vi "HFRR ADV v013 new software.vi"() -> ()   [LabVIEW 2025] (continued)
            frame 2 {
              n1465 = local write "HUMIDITY:"(w1752) -> ()
            }
            frame 3 {
              n1466 = local write "AIR TEMPERATURE :"(w1753) -> ()
            }
            frame 4 {
              n1467 = local write "Com Port 1"(w1754) -> ()
            }
            frame 5 {
              n1468 = local write "Com Port 2"(w1755) -> ()
              n1469 = local write "visa due"(w1755) -> ()
            }
            frame 6 {
              n1470 = String To Path(string=w1756) -> (path=w1757:path)
              n1471 = local write "File Path"(w1757) -> ()
              "String" <- w1756
            }
            frame 7 {
              n1472 = local write "DISPLACEMENT :"(w1758) -> ()
            }
            frame 8 {
              n1473 = local write "STROKE GAIN :"(w1759) -> ()
            }
            frame 9 {
            }
            frame 10 {
              n1474 = local write "Language Selection"(w1760) -> ()
            }
            frame 11 {
              n1475 = local write "CH-POWER +"(w1761) -> ()
            }
            frame 12 {
              n1476 = local write "CH-POWER -"(w1762) -> ()
            }
            frame 13 {
              n1477 = local write "CH-HEATER"(w1763) -> ()
            }
            frame 14 {
              n1478 = local write "CH-HUMIDITY WET"(w1764) -> ()
            }
            frame 15 {
              n1479 = local write "CH-HUMIDITY DRY"(w1765) -> ()
            }
            frame 16 {
            }
            frame 17 {
              n1480 = local write "AIR TEMP INTERCEPT:"(w1766) -> ()
            }
            frame 18 {
              n1481 = local write "TEMP INTERCEPT:"(w1767) -> ()
            }
            frame 21 {
              n1482 = local write "S.NO"(w1768) -> ()
            }
            frame 22 {
              n1483 = local write "Com Port 3"(w1769) -> ()
            }
            frame 20 {
              n1484 = local write "Camera Port :"(w1770) -> ()
            }
            frame 19 {
              n1485 = local write "C3 :"(w1771) -> ()
            }
            frame 23, Default {
            }
          }
        }
      }
    }
    n1486 = Select(t=u32 2500 ("milliseconds to wait"), s=w1724, f=u32 500 ("milliseconds to wait")) -> (s? t:f=w1722:u32)
    n1487 = Multiply(x=w1727, y=w1722) -> (x*y=w1729:dbl)
    n1488 = property on="Time slide" class="Slide (strict)"("Visible"=w1718) -> ()  [unwired: 2 in, 2 out]
    n1489 = call "Elapsed Time2"("Time Target (s)"=w1729, "Auto Reset"=TRUE) -> ("Time has Elapsed"=w1719:bool)  [unwired: 10 in, 7 out]
    n1490 = case shown="True" w1719 {
      frame False {
      }
      frame True {
        n1491 = stacked-sequence {
          frame #0 {
            # "DATA PROCESSING"
            # "115 mV/N"
            n1492 = local read "Sample Temperature"() -> (w1774:dbl)
            n1493 = local read "RH Numeric:"() -> (w1781:dbl)
            n1494 = local read "HUMIDITY:"() -> (w1782:dbl)
            n1495 = local read "FRICVALZ"() -> (w1793:dbl)
            n1496 = local read "Friction"() -> (w1777:dbl)
            n1497 = Multiply(x=w1781, y=w1782) -> (x*y=→"Humidity ( %RH )" →"Hum" →"Hum 2":dbl)
            n1498 = call <vilib>:"Mean PtByPt.vi"("x"=w1774, "sample length"=100) -> ("mean"=w1773:dbl)  [unwired: 2 in, 1 out]
            "TEMP 2" <- w1773
            "TEMP 3" <- w1773
            n1499 = Subtract(x=w1777, y=w1793) -> (x-y=w1788:dbl)
            "FF 2" <- w1788
            "FF 4" <- w1788
            n1500 = local read "Ambient Temperature"() -> (→"AIR TEMP":dbl)
            n1501 = local read "TEMP"() -> (w1792:dbl)
            n1502 = local write "FF 3"(w1788) -> ()
            n1503 = Compound Arithmetic op=OR("FRICVALZ 4", "FRICVALZ 3", "FRICVALZ 2") -> (w1784:bool)
            n1504 = case shown="True" w1784 {
              tunnel: w1777 -> [_ w1799]
              frame False {
              }
              frame True {
                w1798 = FALSE ("FRICVALZ")
                n1505 = local write "FRICVALZ 3"(w1798) -> ()
                n1506 = local write "FRICVALZ 2"(w1798) -> ()
                n1507 = local write "FRICVALZ 4"(w1798) -> ()
                "FRICVALZ" <- w1799
              }
            }
            n1508 = Not A Number/Path/Refnum?(number/path/refnum=w1792) -> (NaN/Path/Refnum?=w1791:bool)
            n1509 = Not A Number/Path/Refnum?(number/path/refnum=w1788) -> (NaN/Path/Refnum?=w1790:bool)
            n1510 = Divide(x=w1788, y=1.96) -> (x/y=w1785:dbl)
            n1511 = Compound Arithmetic op=OR(w1791, w1790) -> (w1789:bool)
            n1512 = Not A Number/Path/Refnum?(number/path/refnum=w1785) -> (NaN/Path/Refnum?=w1786:bool)
            n1513 = case shown="True" w1789 {
              frame False {
              }
              frame True {
                n1514 = local write "TEMP"(0.0 ("TEMP")) -> ()
                n1515 = local write "FF 2"(0.0 ("FF 2")) -> ()
                n1516 = local write "reinit"(TRUE ("reinit")) -> ()
              }
            }
            n1517 = local write "TEMP"(w1773) -> ()
            n1518 = Select(t=0.0, s=w1786, f=w1785) -> (s? t:f=w1776:dbl)
            "COF 2" <- w1776
            n1519 = local write "COF 3"(w1776) -> ()
          }
        }
      }
    }
    n1520 = Wait (ms)(milliseconds to wait=u32 50) -> ()  [unwired: 1 out]
    n1521 = local read "Quit"() -> (w1711:bool)
    "Rate" <- 2500.0 ("No of Samples")
  }
  n1522 = while {
    tunnel: w57 -> [_]
    tunnel: [w1826] -> _
    tunnel: [w1802] -> w56
    i -> [w1826]
    stop <- w1802 stop-if-true
    # "C:\\LAB-IQ-NXT\\Scar View.exe"
    n1523 = local read "OK Button 16"() -> (w1815:bool)
    n1524 = local read "Main Tab"() -> (w1808:T2)
    n1525 = local read "service 3"() -> (w1809:bool)
    n1526 = local read "OPEN 6"() -> (w1811:bool)
    n1527 = local read "EDIT 2"() -> (w1813:bool)
    n1528 = flat-sequence {
      frame #0 {
        n1529 = local read "SAVE 2"() -> (w2428:bool)
        n1530 = stacked-sequence {
          frame #0 {
            n1531 = local read "EDIT"() -> (w2482:bool)
            n1532 = case shown="True" w2482 {
              tunnel: [u8 2 ("Disabled") u8 0 ("Disabled")] -> _
              frame False {
                w2484 = FALSE
                n1533 = local write "Password"("") -> ()
                n1534 = property on="SrvM CP" class="Bool (strict)"("Visible"=w2484) -> ()  [unwired: 2 in, 2 out]
                n1535 = property on="message" class="Str"("Visible"=w2484) -> ()  [unwired: 2 in, 2 out]
                n1536 = local write "x = y?"(w2484) -> ()
                n1537 = property on="Password" class="Str"("Visible"=w2484) -> ()  [unwired: 2 in, 2 out]
                n1538 = property on="ENTER THE NEW PASSWORD" class="Str"("Visible"=w2484) -> ()  [unwired: 2 in, 2 out]
                n1539 = property on="ENTER CURRENT PASSWORD" class="Str"("Visible"=w2484) -> ()  [unwired: 2 in, 2 out]
                n1540 = local write "SrvM CP"(w2484) -> ()
              }
              frame True {
                w2487 = TRUE
                n1541 = property on="SrvM CP" class="Bool (strict)"("Visible"=w2487) -> ()  [unwired: 2 in, 2 out]
                n1542 = property on="Password" class="Str"("Visible"=w2487) -> ()  [unwired: 2 in, 2 out]
              }
            }
            "dipl pwd" <- "@143$\n" ("dipl pwd")
          }
          frame #1 {
            # "Gain password"
            n1543 = String To Byte Array(string="ENTER CURRENT PASSWORD") -> (unsigned byte array=w2492:u8[])
            n1544 = Search 1D Array(1D array=w2492, element=u8 10) -> (index of element=w2495:i32)  [unwired: 1 in]
            n1545 = Index Array(array=w2492, index=w2495) -> (element=w2491:u8)
            n1546 = Equal?(x=w2491, y=10) -> (x = y?=w2489:bool)
            n1547 = case shown="True" w2489 {
              frame False {
                n1548 = property on="ENTER THE NEW PASSWORD" class="Str"("Visible"=FALSE) -> ()  [unwired: 2 in, 2 out]
              }
              frame True {
                # "password"
                # "change password logic"
                n1549 = local read "ENTER CURRENT PASSWORD"() -> (w2508:string)
                n1550 = local read "dipl pwd"() -> (w2502:string)
                n1551 = String To Byte Array(string=w2508) -> (unsigned byte array=w2510:u8[])
                n1552 = String To Byte Array(string=w2502) -> (unsigned byte array=w2503:u8[])
                n1553 = Array Size(array=w2510) -> (size(s)=w2507:i32)
                n1554 = Array Size(array=w2503) -> (size(s)=w2505:i32)
                n1555 = for {
                  N: w2507 -> [_]
                  tunnel: w2510 -> [w2534]
                  tunnel: [w2532] -> w2511 mode=indexing
                  tunnel: w2507 -> [w2526]
                  i -> [w2527]
                  n1556 = Decrement(x=w2526) -> (x-1=w2524:i32)
                  n1557 = Equal?(x=w2527, y=w2524) -> (x = y?=w2525:bool)
                  n1558 = Index Array(array=w2534, index=w2527) -> (element=w2528:u8)
                  n1559 = Number To Decimal String(number=w2528) -> (decimal integer string=w2533:string)  [unwired: 1 in]
                  n1560 = Select(t="", s=w2525, f="\r") -> (s? t:f=w2530:string)
                  n1561 = Concatenate Strings(w2533, w2530) -> (w2532:string)
                }
                n1562 = for {
                  N: w2505 -> [_]
                  tunnel: w2503 -> [w2522]
                  tunnel: [w2520] -> w2504 mode=indexing
                  tunnel: w2505 -> [w2517]
                  i -> [w2518]
                  n1563 = Decrement(x=w2517) -> (x-1=w2516:i32)
                  n1564 = Equal?(x=w2518, y=w2516) -> (x = y?=w2515:bool)
                  n1565 = Index Array(array=w2522, index=w2518) -> (element=w2521:u8)
                  n1566 = Number To Decimal String(number=w2521) -> (decimal integer string=w2519:string)  [unwired: 1 in]
                  n1567 = Select(t="", s=w2515, f="\r") -> (s? t:f=w2512:string)
                  n1568 = Concatenate Strings(w2519, w2512) -> (w2520:string)
                }
                n1569 = local read "string"() -> (w2509:string)
                n1570 = Concatenate Strings(w2504) -> (w2498:string)
                n1571 = Concatenate Strings(w2509) -> (w2506:string)
                n1572 = Concatenate Strings(w2511) -> (w2499:string)
                n1573 = Equal?(x=w2499, y=w2506) -> (x = y?=w2501:bool)
                n1574 = Equal?(x=w2499, y=w2498) -> (x = y?=w2497:bool)
                n1575 = Or(x=w2501, y=w2497) -> (x .or. y?=w2500:bool)
                n1576 = case shown="True" w2500 {
                  frame False {
                  }
                  frame True {
                    n1577 = property on="ENTER THE NEW PASSWORD" class="Str"("Visible"=TRUE) -> ()  [unwired: 2 in, 2 out]
                  }
                }
              }
            }
          }
          frame #2 {
            n1578 = String To Byte Array(string="ENTER THE NEW PASSWORD") -> (unsigned byte array=w2537:u8[])
            n1579 = Search 1D Array(1D array=w2537, element=u8 10) -> (index of element=w2541:i32)  [unwired: 1 in]
            n1580 = Index Array(array=w2537, index=w2541) -> (element=w2539:u8)
            n1581 = Equal?(x=w2539, y=10) -> (x = y?=w2536:bool)
            n1582 = case shown="False" w2536 {
              frame False {
              }
              frame True {
                n1583 = local write "EDIT"(FALSE) -> ()
                n1584 = local write "SrvM CP"(FALSE) -> ()
                n1585 = local read "ENTER THE NEW PASSWORD"() -> (w2544:string)
                n1586 = String To Byte Array(string=w2544) -> (unsigned byte array=w2549:u8[])
                n1587 = Array Size(array=w2549) -> (size(s)=w2546:i32)
                n1588 = for {
                  N: w2546 -> [_]
                  tunnel: w2549 -> [w2562]
                  tunnel: [w2559] -> w2551 mode=indexing
                  tunnel: w2546 -> [w2554]
                  i -> [w2552]
                  n1589 = Decrement(x=w2554) -> (x-1=w2555:i32)
                  n1590 = Equal?(x=w2552, y=w2555) -> (x = y?=w2556:bool)
                  n1591 = Index Array(array=w2562, index=w2552) -> (element=w2561:u8)
                  n1592 = Number To Decimal String(number=w2561) -> (decimal integer string=w2560:string)  [unwired: 1 in]
                  n1593 = Select(t="", s=w2556, f="\r") -> (s? t:f=w2553:string)
                  n1594 = Concatenate Strings(w2560, w2553) -> (w2559:string)
                }
                n1595 = local read "file path"() -> (w2543:path)
                n1596 = Concatenate Strings(w2551) -> (w2545:string)
                n1597 = Delete(path (use dialog)=w2543) -> (deleted path=w2547:path)  [unwired: 4 in, 2 out]
                n1598 = call <vilib>:"Write Characters To File.vi"("append to file? (new file:F)"=FALSE, "character string"=w2545, "file path (dialog if empty)"=w2547) -> ()  [unwired: 2 in, 1 out]
              }
            }
          }
          frame #3 {
            n1599 = case shown="True" "SrvM CP" {
              frame False {
                w2565 = ""
                n1600 = local write "ENTER CURRENT PASSWORD"(w2565) -> ()
                n1601 = local write "ENTER THE NEW PASSWORD"(w2565) -> ()
                n1602 = property on="ENTER CURRENT PASSWORD" class="Str"("Visible"=FALSE) -> ()  [unwired: 2 in, 2 out]
              }
              frame True {
                n1603 = property on="ENTER THE NEW PASSWORD" class="Str"() -> ("Visible"=w2566:bool)  [unwired: 2 in, 2 out]
                n1604 = Not(x=w2566) -> (.not. x?=w2567:bool)
                n1605 = property on="ENTER CURRENT PASSWORD" class="Str"("Visible"=w2567) -> ()  [unwired: 2 in, 2 out]
              }
            }
          }
          frame #4 {
            n1606 = String To Byte Array(string="Password") -> (unsigned byte array=w2574:u8[])
            n1607 = Search 1D Array(1D array=w2574, element=u8 10) -> (index of element=w2572:i32)  [unwired: 1 in]
            n1608 = Index Array(array=w2574, index=w2572) -> (element=w2573:u8)
            n1609 = Equal?(x=w2573, y=10) -> (x = y?=w2569:bool)
            n1610 = case shown="True" w2569 {
              frame False {
              }
              frame True {
                # "password"
                # "password"
                n1611 = local read "Password"() -> (w2587:string)
                n1612 = String To Byte Array(string=w2587) -> (unsigned byte array=w2590:u8[])
                n1613 = String To Byte Array(string="@143$\n") -> (unsigned byte array=w2576:u8[])
                n1614 = Array Size(array=w2590) -> (size(s)=w2585:i32)
                n1615 = Array Size(array=w2576) -> (size(s)=w2581:i32)
                n1616 = for {
                  N: w2585 -> [_]
                  tunnel: w2590 -> [w2624]
                  tunnel: [w2622] -> w2591 mode=indexing
                  tunnel: w2585 -> [w2619]
                  i -> [w2620]
                  n1617 = Decrement(x=w2619) -> (x-1=w2618:i32)
                  n1618 = Index Array(array=w2624, index=w2620) -> (element=w2623:u8)
                  n1619 = Equal?(x=w2620, y=w2618) -> (x = y?=w2617:bool)
                  n1620 = Number To Decimal String(number=w2623) -> (decimal integer string=w2621:string)  [unwired: 1 in]
                  n1621 = Select(t="", s=w2617, f="\r") -> (s? t:f=w2614:string)
                  n1622 = Concatenate Strings(w2621, w2614) -> (w2622:string)
                }
                n1623 = for {
                  N: w2581 -> [_]
                  tunnel: w2576 -> [w2635]
                  tunnel: [w2633] -> w2579 mode=indexing
                  tunnel: w2581 -> [w2630]
                  i -> [w2631]
                  n1624 = Decrement(x=w2630) -> (x-1=w2629:i32)
                  n1625 = Index Array(array=w2635, index=w2631) -> (element=w2634:u8)
                  n1626 = Equal?(x=w2631, y=w2629) -> (x = y?=w2628:bool)
                  n1627 = Number To Decimal String(number=w2634) -> (decimal integer string=w2632:string)  [unwired: 1 in]
                  n1628 = Select(t="", s=w2628, f="\r") -> (s? t:f=w2625:string)
                  n1629 = Concatenate Strings(w2632, w2625) -> (w2633:string)
                }
                n1630 = local read "file path"() -> (w2575:path)
                n1631 = call <vilib>:"Read Characters From File.vi"("file path (dialog if empty)"=w2575) -> ("character string"=w2589:string)  [unwired: 5 in, 3 out]
                "string" <- w2589
                n1632 = flat-sequence {
                  tunnel: [w2592] -> w2586
                  frame #0 {
                    w2592 = ""
                    n1633 = local write "Password"(w2592) -> ()
                  }
                }
                n1634 = Concatenate Strings(w2579) -> (w2580:string)
                n1635 = Concatenate Strings(w2589) -> (w2588:string)
                n1636 = Concatenate Strings(w2591) -> (w2583:string)
                n1637 = Equal?(x=w2583, y=w2588) -> (x = y?=w2578:bool)
                n1638 = Equal?(x=w2583, y=w2580) -> (x = y?=w2584:bool)
                n1639 = Or(x=w2578, y=w2584) -> (x .or. y?=w2577:bool)
                "x = y?" <- w2577
                n1640 = case shown="True" w2577 {
                  selector: w2577 -> [w2594 _]
                  tunnel: w2586 -> [_ _]
                  frame False {
                    n1641 = And(x=w2594, y=TRUE ("Visible")) -> (x .and. y?=w2595:bool)
                    n1642 = property on="message" class="Str"("Visible"=w2595) -> ()  [unwired: 2 in, 2 out]
                  }
                  frame True {
                    n1643 = control-ref of="This VI"() -> (w2606:refnum<vi>)
                    n1644 = property class="VI"(reference=w2606) -> (reference out=w2597:refnum<vi>, error out=w2601:errorcluster, "Panel"=w2605:refnum<vi>)  [unwired: 1 in]
                    n1645 = property on="message" class="Str"("Visible"=FALSE) -> ()  [unwired: 2 in, 2 out]
                    n1646 = property class="Pnl"(reference=w2605, error in=w2601) -> (reference out=w2599:refnum<vi>, error out=w2602:errorcluster, "Panes[]"=w2604:refnum<vi>[])
                    n1647 = for {
                      tunnel: w2604 -> [w2613] mode=indexing
                      tunnel: T20."Always On" ("Horizontal Scrollbar Visibility") -> [w2612]
                      tunnel: w2602 -> [w2609]
                      tunnel: [w2608] -> w2600
                      n1648 = property class="Pane"(reference=w2613, error in=w2609, "HorizScrollbarVisibility"=w2612) -> (reference out=w2610:refnum<vi>, error out=w2611:errorcluster)
                      n1649 = Close Reference(reference=w2610, error in (no error)=w2611) -> (error out=w2608:errorcluster)
                    }
                    n1650 = Close Reference(reference=w2599, error in (no error)=w2600) -> (error out=w2598:errorcluster)
                    n1651 = Close Reference(reference=w2597, error in (no error)=w2598) -> (error out=→"error out 6":errorcluster)
                  }
                }
              }
            }
          }
        }
        n1652 = local read "x = y?"() -> (w2434:bool)
        n1653 = local read "HUMIDITY: 2"() -> (w2436:dbl)
        n1654 = local read "HUMIDITY:"() -> (w2435:dbl)
        n1655 = property on="Port 2 Error" class="Clust (strict)"("Visible"="EDIT") -> ()  [unwired: 2 in, 2 out]
        n1656 = property on="Port 1 Error" class="Clust (strict)"("Visible"="EDIT") -> ()  [unwired: 2 in, 2 out]
        n1657 = case shown="True" "SrvM CP 2" {
          frame False {
          }
          frame True {
            n1658 = local write "SrvM CP 2"(FALSE ("SrvM CP 2")) -> ()
            n1659 = local read "HUMIDITY: 2"() -> (w2475:dbl)
            n1660 = local read "TEMP INTERCEPT: 2"() -> (w2474:dbl)
            n1661 = local read "DISPLACEMENT : 4"() -> (w2478:dbl)
            n1662 = local read "TEMPERATURE : 2"() -> (w2477:dbl)
            n1663 = local read "STROKE GAIN : 2"() -> (w2479:dbl)
            n1664 = local read "FRIC. FORCE : 2"() -> (w2480:dbl)
            n1665 = local read "AIR TEMP INTERCEPT: 2"() -> (w2473:dbl)
            n1666 = local read "AIR TEMPERATURE : 2"() -> (w2476:dbl)
            n1667 = local write "HUMIDITY:"(w2475) -> ()
            n1668 = local write "AIR TEMP INTERCEPT:"(w2474) -> ()
            n1669 = local write "TEMPERATURE :"(w2477) -> ()
            n1670 = local write "FRIC. FORCE :"(w2480) -> ()
            n1671 = local write "STROKE GAIN :"(w2479) -> ()
            n1672 = local write "DISPLACEMENT :"(w2478) -> ()
            n1673 = local write "AIR TEMPERATURE :"(w2476) -> ()
            n1674 = local write "TEMP INTERCEPT:"(w2473) -> ()
          }
        }
        n1675 = Or(x="SAVE", y=w2428) -> (x .or. y?=w2429:bool)
        n1676 = And(x="EDIT", y=w2434) -> (x .and. y?=w2432:bool)
        n1677 = local read "DISPLACEMENT : 4"() -> (w2445:dbl)
        n1678 = local read "TEMPERATURE : 2"() -> (w2443:dbl)
        n1679 = local read "STROKE GAIN : 2"() -> (w2449:dbl)
        n1680 = local read "DISPLACEMENT :"() -> (w2444:dbl)
        n1681 = local read "FRIC. FORCE : 2"() -> (w2452:dbl)
        n1682 = local read "TEMPERATURE :"() -> (w2441:dbl)
        n1683 = local read "STROKE GAIN :"() -> (w2448:dbl)
        n1684 = local read "FRIC. FORCE :"() -> (w2451:dbl)
        n1685 = case shown="True" w2432 {
          tunnel: [u8 2 ("Disabled") u8 0 ("Disabled")] -> w2431
          tunnel: [w2796 TRUE ("Visible")] -> w2430
          frame False {
            w2796 = FALSE ("Visible")
            n1686 = local write "EDIT 2"(w2796) -> ()
          }
          frame True {
          }
        }
        n1687 = case shown="True" w2429 {
          frame False {
          }
          frame True {
            n1688 = stacked-sequence {
              seq-local: [w2644 _ _] -> [_ w2791 _]
              frame #0 {
                (unwired) i16 5 ("precision (6)")
                # "[CH1]    - FF\n[CH2]   - TEMPERATURE\n[CH3]    - Humidity\n[CH4]    - AIR TEMP\n[CH5]\\- Visa Uno\n[CH6] \\- Visa Due\n[CH7]  \\- file path\n[CH8]   - Displacement Gain\n[CHA]   - Stroke Gain\n[CHB]   - Stroke PID Gain\n[CHC]   -Language Selection\n[CHD]   -Power +\n[CHE]   -Power_\n[CHF]   -Heater\n[CHG]   -Humidity Wet\n[CHH]   -Humidity Dry\n[CHI]   -Integral Time"
                n1689 = local read "Language Selection"() -> (w2692:enum16{"English", "Russian"})
                n1690 = local read "CH-HUMIDITY WET"() -> (w2650:u16)
                n1691 = local read "CH-HUMIDITY DRY"() -> (w2647:u16)
                n1692 = local read "STROKE GAIN :"() -> (w2636:dbl)
                n1693 = local read "CH-POWER +"() -> (w2659:u16)
                n1694 = local read "CH-POWER -"() -> (w2656:u16)
                n1695 = local read "CH-HEATER"() -> (w2653:u16)
                n1696 = local read "AIR TEMPERATURE :"() -> (w2639:dbl)
                n1697 = local read "DISPLACEMENT :"() -> (w2637:dbl)
                n1698 = local read "TEMPERATURE :"() -> (w2640:dbl)
                n1699 = local read "FRIC. FORCE :"() -> (w2641:dbl)
                n1700 = local read "HUMIDITY:"() -> (w2638:dbl)
                n1701 = Path To String(path="File Path") -> (string=w2708:string)
                n1702 = Number To Fractional String(number=w2636, width (-)=i16 10 ("precision (6)"), precision (6)=i16 5) -> (F-format string=w2699:string)  [unwired: 1 in]
                n1703 = Number To Fractional String(number=w2692, width (-)=i16 10 ("precision (6)"), precision (6)=i16 5) -> (F-format string=w2688:string)  [unwired: 1 in]
                n1704 = Number To Fractional String(number=w2659, width (-)=i16 10 ("precision (6)"), precision (6)=i16 5) -> (F-format string=w2682:string)  [unwired: 1 in]
                n1705 = Number To Fractional String(number=w2656, width (-)=i16 10 ("precision (6)"), precision (6)=i16 5) -> (F-format string=w2679:string)  [unwired: 1 in]
                n1706 = Number To Fractional String(number=w2653, width (-)=i16 10 ("precision (6)"), precision (6)=i16 5) -> (F-format string=w2674:string)  [unwired: 1 in]
                n1707 = Number To Fractional String(number=w2650, width (-)=i16 10 ("precision (6)"), precision (6)=i16 5) -> (F-format string=w2671:string)  [unwired: 1 in]
                n1708 = Number To Fractional String(number=w2647, width (-)=i16 10 ("precision (6)"), precision (6)=i16 5) -> (F-format string=w2666:string)  [unwired: 1 in]
                n1709 = local read "Com Port 1"() -> (w2643:refnum<visa-resource-name>)
                n1710 = local read "Com Port 2"() -> (w2642:refnum<visa-resource-name>)
                n1711 = Concatenate Strings(w2708, "\\" ("string")) -> (w2707:string)
                n1712 = Number To Fractional String(number=w2641, width (-)=i16 10 ("precision (6)"), precision (6)=i16 5) -> (F-format string=w2740:string)  [unwired: 1 in]
                n1713 = Number To Fractional String(number=w2640, width (-)=i16 10 ("precision (6)"), precision (6)=i16 5) -> (F-format string=w2739:string)  [unwired: 1 in]
                n1714 = Number To Fractional String(number=w2638, width (-)=i16 10 ("precision (6)"), precision (6)=i16 5) -> (F-format string=w2733:string)  [unwired: 1 in]
                n1715 = Number To Fractional String(number=w2639, width (-)=i16 10 ("precision (6)"), precision (6)=i16 5) -> (F-format string=w2727:string)  [unwired: 1 in]
                n1716 = Number To Fractional String(number=w2637, width (-)=i16 10 ("precision (6)"), precision (6)=i16 5) -> (F-format string=w2700:string)  [unwired: 1 in]
                n1717 = Concatenate Strings("[CHA]" ("string"), w2699, "- Stroke Gain" ("string"), "\r") -> (w2693:string)
                n1718 = Concatenate Strings("[CHC]" ("string"), w2688, "-Language Selection" ("string"), "\r") -> (w2685:string)
                n1719 = Concatenate Strings("[CHD]" ("string"), w2682, "-Power +" ("string"), "\r") -> (w2664:string)
                n1720 = Concatenate Strings("[CHG]" ("string"), w2671, "-Humidity Wet" ("string"), "\r") -> (w2661:string)
                n1721 = Concatenate Strings("[CHH]" ("string"), w2666, "-Humidity Dry" ("string"), "\r") -> (w2660:string)
                n1722 = Concatenate Strings("[CH1]" ("string"), w2740, " - FF" ("string"), "\r") -> (w2738:string)
                n1723 = Concatenate Strings("[CH2]" ("string"), w2739, " - TEMPERATURE" ("string"), "\r") -> (w2737:string)
                n1724 = Concatenate Strings("[CH3]" ("string"), w2733, " - Humidity" ("string"), "\r") -> (w2730:string)
                n1725 = Concatenate Strings("[CH4]" ("string"), w2727, " - AIR TEMP" ("string"), "\r") -> (w2723:string)
                n1726 = Concatenate Strings("[CH5]" ("string"), w2643, "- Visa Uno" ("string"), "\r") -> (w2716:string)
                n1727 = Concatenate Strings("[CH6]" ("string"), w2642, "- Visa Due" ("string"), "\r") -> (w2711:string)
                n1728 = Concatenate Strings("[CH7]" ("string"), w2707, "- file path" ("string"), "\r") -> (w2710:string)
                n1729 = Concatenate Strings("[CH8]" ("string"), w2700, "- Displacement Gain" ("string"), "\r") -> (w2703:string)
                n1730 = Concatenate Strings("[CHE]" ("string"), w2679, "-Power_" ("string"), "\r") -> (w2663:string)
                n1731 = Concatenate Strings("[CHF]" ("string"), w2674, "-Heater" ("string"), "\r") -> (w2662:string)
                n1732 = Concatenate Strings(w2738, w2737, w2730, w2723, w2716, w2711, w2710, w2703, w2693, w2685, w2664, w2663, w2662, w2661, w2660) -> (w2644:string)
                "gain" <- w2644
              }
              frame #1 {
                n1733 = local read "Camera Port :"() -> (w2752:string)
                n1734 = local read "C3 :"() -> (w2760:refnum<visa-resource-name>)
                n1735 = local read "TEMP INTERCEPT:"() -> (w2761:dbl)
                n1736 = local read "AIR TEMP INTERCEPT:"() -> (w2762:dbl)
                n1737 = local read "Com Port 3"() -> (w2763:refnum<visa-resource-name>)
                n1738 = Concatenate Strings("[CH8]" ("string"), w2752, "- Visa Camera" ("string"), "\r") -> (w2751:string)
                n1739 = Concatenate Strings("[CH7]" ("string"), w2760, "- Visa Humidity" ("string"), "\r") -> (w2756:string)
                n1740 = Number To Fractional String(number=w2761, width (-)=i16 10 ("precision (6)"), precision (6)=i16 5) -> (F-format string=w2779:string)  [unwired: 1 in]
                n1741 = Concatenate Strings("[CHL]" ("string"), w2763, "- Visa humid" ("string"), "\r") -> (w2766:string)
                n1742 = Number To Fractional String(number=w2762, width (-)=i16 10 ("precision (6)"), precision (6)=i16 5) -> (F-format string=w2786:string)  [unwired: 1 in]
                n1743 = Concatenate Strings("[CHK]" ("string"), w2779, "-TEMP INTERCEPT" ("string"), "\r") -> (w2775:string)
                n1744 = Concatenate Strings("[SNO]" ("string"), "S.NO", "-" ("string"), "\r") -> (w2771:string)
                n1745 = Concatenate Strings("[CHJ]" ("string"), w2786, "-AIR TEMP INTERCEPT" ("string"), "\r") -> (w2776:string)
                n1746 = String To Path(string="C:\\LAB-IQ\\calibrate WO 2465.dcf") -> (path=w2764:path)
                n1747 = Concatenate Strings(w2791, w2776, w2775, w2771, w2766, w2756, w2751) -> (w2790:string)
                n1748 = call <vilib>:"Write Characters To File.vi"("append to file? (new file:F)"=FALSE, "character string"=w2790, "file path (dialog if empty)"=w2764) -> ()  [unwired: 2 in, 1 out]
              }
              frame #2 {
                n1749 = local write "Lan flag"(0.0 ("Lan flag")) -> ()
                n1750 = local write "conststatus"(0.0 ("rpm value : 2")) -> ()
                n1751 = local write "SAVE"(FALSE ("OK Button 14")) -> ()
                n1752 = local write "SAVE 2"(FALSE ("SAVE 2")) -> ()
              }
            }
          }
        }
        n1753 = Subtract(x=w2436, y=w2435) -> (x-y=w2437:dbl)
        n1754 = local read "AIR TEMPERATURE : 2"() -> (w2440:dbl)
        n1755 = local read "AIR TEMPERATURE :"() -> (w2439:dbl)
        n1756 = Divide(x=w2437, y=w2435) -> (x/y=w2459:dbl)
        n1757 = Subtract(x=w2452, y=w2451) -> (x-y=w2450:dbl)
        n1758 = Subtract(x=w2443, y=w2441) -> (x-y=w2442:dbl)
        n1759 = Subtract(x=w2449, y=w2448) -> (x-y=w2447:dbl)
        n1760 = Subtract(x=w2445, y=w2444) -> (x-y=w2446:dbl)
        n1761 = Subtract(x=w2440, y=w2439) -> (x-y=w2438:dbl)
        n1762 = Divide(x=w2450, y=w2451) -> (x/y=w2470:dbl)
        n1763 = Divide(x=w2442, y=w2441) -> (x/y=w2463:dbl)
        n1764 = Divide(x=w2447, y=w2448) -> (x/y=w2467:dbl)
        n1765 = Divide(x=w2446, y=w2444) -> (x/y=w2466:dbl)
        n1766 = Multiply(x=w2459, y=100.0) -> (x*y=→"HUMIDITY  Calibration Error":dbl)
        n1767 = Divide(x=w2438, y=w2439) -> (x/y=w2462:dbl)
        n1768 = Multiply(x=w2470, y=100.0) -> (x*y=→"FRIC. FORCE Calibration Error":dbl)
        n1769 = Multiply(x=w2463, y=100.0) -> (x*y=→"TEMPERATURE  Calibration Error":dbl)
        n1770 = Multiply(x=w2467, y=100.0) -> (x*y=→"STROKE Calibration Error":dbl)
        n1771 = Multiply(x=w2466, y=100.0) -> (x*y=→"DISPLACEMENT  Calibration Error":dbl)
        n1772 = property on="EDIT 2" class="Bool (strict)"("Visible"=w2430) -> ()  [unwired: 2 in, 2 out]
        n1773 = property on="SAVE" class="Bool (strict)"("Visible"=w2430) -> ()  [unwired: 2 in, 2 out]
        n1774 = property on="SrvM CP" class="Bool (strict)"("Disabled"=w2431) -> ()  [unwired: 2 in, 2 out]
        n1775 = property on="visa due" class="CmbBox"("Disabled"=w2431) -> ()  [unwired: 2 in, 2 out]
        n1776 = property on="File Path" class="Path"("Disabled"=w2431) -> ()  [unwired: 2 in, 2 out]
        n1777 = Multiply(x=w2462, y=100.0) -> (x*y=→"AIR TEMPERATURE  Calibration Error":dbl)
        n1778 = property on="Language Selection" class="Enum (strict)"("Visible"=w2430) -> ()  [unwired: 2 in, 2 out]
        n1779 = property on="Tab Control 7" class="TabCtl (strict)"("Disabled"=w2431) -> ()  [unwired: 2 in, 2 out]
        n1780 = property on="AIR TEMP INTERCEPT:" class="DigNum (strict)"("Disabled"=w2431) -> ()  [unwired: 2 in, 2 out]
        n1781 = property on="CH-POWER -" class="DigNum (strict)"("Disabled"=w2431) -> ()  [unwired: 2 in, 2 out]
        n1782 = property on="CH-POWER +" class="DigNum (strict)"("Disabled"=w2431) -> ()  [unwired: 2 in, 2 out]
        n1783 = property on="AIR TEMPERATURE :" class="DigNum (strict)"("Disabled"=w2431) -> ()  [unwired: 2 in, 2 out]
        n1784 = property on="STROKE GAIN :" class="DigNum (strict)"("Disabled"=w2431) -> ()  [unwired: 2 in, 2 out]
        n1785 = property on="SPEED OUT:" class="DigNum (strict)"("Disabled"=w2431) -> ()  [unwired: 2 in, 2 out]
        n1786 = property on="CH-HUMIDITY DRY" class="DigNum (strict)"("Disabled"=w2431) -> ()  [unwired: 2 in, 2 out]
        n1787 = property on="HUMIDITY:" class="DigNum (strict)"("Disabled"=w2431) -> ()  [unwired: 2 in, 2 out]
        n1788 = property on="CH-HUMIDITY WET" class="DigNum (strict)"("Disabled"=w2431) -> ()  [unwired: 2 in, 2 out]
        n1789 = property on="TEMPERATURE :" class="DigNum (strict)"("Disabled"=w2431) -> ()  [unwired: 2 in, 2 out]
        n1790 = property on="DISPLACEMENT :" class="DigNum (strict)"("Disabled"=w2431) -> ()  [unwired: 2 in, 2 out]
        n1791 = property on="CH-HEATER" class="DigNum (strict)"("Disabled"=w2431) -> ()  [unwired: 2 in, 2 out]
        n1792 = property on="TEMP INTERCEPT:" class="DigNum (strict)"("Disabled"=w2431) -> ()  [unwired: 2 in, 2 out]
        n1793 = property on="FRIC. FORCE :" class="DigNum (strict)"("Disabled"=w2431) -> ()  [unwired: 2 in, 2 out]
      }
    }
    n1794 = local read "RUN"() -> (w1825:bool)
    n1795 = local read "RUN"() -> (w1823:bool)
    n1796 = disable-structure shown="Disabled" {
      disable-tunnel: [w1840 _] -> w1806
      disable-tunnel: [w1839 _] -> w1804
      frame Disabled {
        n1797 = local read "Temperature before test"() -> (w1833:dbl)
        n1798 = local read "Temperature after test"() -> (w1846:dbl)
        n1799 = case shown="True" "Save Results" {
          frame False {
          }
          frame True {
            w1862 = "\r"
            n1800 = local write "Save Results"(FALSE ("OK Button 5")) -> ()
            n1801 = local read "Temperature before test"() -> (w1900:dbl)
            n1802 = local read "Temperature after test"() -> (w1902:dbl)
            n1803 = local read "Humidity before test"() -> (w1899:dbl)
            n1804 = local read "Humidity after test"() -> (w1901:dbl)
            n1805 = local read "WS1.4"() -> (w1906:dbl)
            n1806 = local read "AVP"() -> (w1904:dbl)
            n1807 = Number To Fractional String(number=w1906, width (-)=i16 6, precision (6)=i16 1) -> (F-format string=w1866:string)  [unwired: 1 in]
            n1808 = local read "MWSD"() -> (w1903:dbl)
            n1809 = local read "String"() -> (w1895:string)
            n1810 = local read "FILE"() -> (w1898:string)
            n1811 = local read "HCF"() -> (w1905:dbl)
            n1812 = Number To Fractional String(number=w1899, width (-)=i16 6, precision (6)=i16 1) -> (F-format string=w1891:string)  [unwired: 1 in]
            n1813 = Number To Fractional String(number=w1900, width (-)=i16 6, precision (6)=i16 1) -> (F-format string=w1888:string)  [unwired: 1 in]
            n1814 = Number To Fractional String(number=w1901, width (-)=i16 6, precision (6)=i16 1) -> (F-format string=w1884:string)  [unwired: 1 in]
            n1815 = Number To Fractional String(number=w1902, width (-)=i16 6, precision (6)=i16 1) -> (F-format string=w1880:string)  [unwired: 1 in]
            n1816 = Number To Fractional String(number=w1904, width (-)=i16 6, precision (6)=i16 3) -> (F-format string=w1873:string)  [unwired: 1 in]
            n1817 = Concatenate Strings(w1895, w1898) -> (w1917:string)
            n1818 = Number To Fractional String(number=w1903, width (-)=i16 6, precision (6)=i16 1) -> (F-format string=w1877:string)  [unwired: 1 in]
            n1819 = Number To Fractional String(number=w1905, width (-)=i16 6, precision (6)=i16 2) -> (F-format string=w1871:string)  [unwired: 1 in]
            n1820 = Concatenate Strings("(" ("string"), w1866, ")Microns" ("string")) -> (w1865:string)
            n1821 = local read "REMARKS"() -> (w1897:string)
            "REMARKS 2" <- w1897
            n1822 = Concatenate Strings("(" ("string"), w1891, " ) % RH," ("string")) -> (w1892:string)
            n1823 = Concatenate Strings(w1871, ")" ("string")) -> (w1869:string)
            n1824 = Concatenate Strings("(" ("string"), w1888, ")  Deg C ," ("string")) -> (w1887:string)
            n1825 = Concatenate Strings("(" ("string"), w1884, " ) % RH," ("string")) -> (w1883:string)
            n1826 = Concatenate Strings("(" ("string"), w1880, ")  Deg C ," ("string")) -> (w1879:string)
            n1827 = Concatenate Strings("(" ("string"), w1877, ")  Microns," ("string")) -> (w1876:string)
            n1828 = Concatenate Strings("(" ("string"), w1873, ")  kPa," ("string")) -> (w1863:string)
            n1829 = Concatenate Strings(w1917, ".dwm" ("Substring")) -> (w1915:string)
            n1830 = String To Path(string=w1915) -> (path=w1914:path)
            n1831 = Concatenate Strings(w1897, w1862, " Humidity before test= " ("Substring"), w1892, w1862, " Temperature before test = " ("Substring"), w1887, w1862, " Humidity after test= " ("Substring"), w1883, w1862, "Temperature after test = " ("Substring"), w1879, w1862, "MSD = " ("Substring"), w1876, w1862, "  AVP = " ("Substring"), w1863, w1862, "  HCF                     =( " ("Substring"), w1869, w1862, " WS1.4                  = " ("Substring"), w1865, w1862) -> (w1861:string)
            "data" <- w1861
            n1832 = call <vilib>:"Write Characters To File.vi"("append to file? (new file:F)"=FALSE, "character string"=w1861, "file path (dialog if empty)"=w1914) -> ()  [unwired: 2 in, 1 out]
            n1833 = Match Pattern(string=w1861, regular expression="!") -> (after substring=→"export":string)  [unwired: 1 in, 3 out]
          }
        }
        n1834 = Add(x=231.864, y=w1833) -> (x+y=w1830:dbl)
        n1835 = Add(x=231.864, y=w1846) -> (x+y=w1843:dbl)
        n1836 = Divide(x=1705.984, y=w1830) -> (x/y=w1831:dbl)
        n1837 = Divide(x=1705.984, y=w1843) -> (x/y=w1844:dbl)
        n1838 = local read "Humidity before test"() -> (w1835:dbl)
        n1839 = local read "Humidity after test"() -> (w1848:dbl)
        n1840 = Subtract(x=8.017352 ("y"), y=w1831) -> (x-y=w1857:dbl)
        n1841 = Subtract(x=8.017352 ("y"), y=w1844) -> (x-y=w1851:dbl)
        n1842 = expression code="10**y"(w1857) -> (w1837:dbl)
        n1843 = expression code="10**y"(w1851) -> (w1850:dbl)
        n1844 = Multiply(x=w1835, y=w1837) -> (x*y=w1836:dbl)
        n1845 = Multiply(x=w1848, y=w1850) -> (x*y=w1849:dbl)
        n1846 = Divide(x=w1836, y=750.0) -> (x/y=w1852:dbl)
        n1847 = Divide(x=w1849, y=750.0) -> (x/y=w1853:dbl)
        n1848 = Add(x=w1852, y=w1853) -> (x+y=w1854:dbl)
        n1849 = Divide(x=w1854, y=2.0) -> (x/y=w1856:dbl)
        n1850 = local write "AVP"(w1856) -> ()
        n1851 = Subtract(x=1.4, y=w1856) -> (x-y=w1839:dbl)
        n1852 = local read "HCF"() -> (w1840:dbl)
      }
      frame Enabled {
      }
    }
    n1853 = case shown="True" "EDIT 3" {
      frame False {
      }
      frame True {
        n1854 = local write "EDIT 3"(FALSE ("EDIT 3")) -> ()
        n1855 = local write "Main Tab"(T2."About" ("Main Tab")) -> ()
      }
    }
    n1856 = case shown="False" w1825 {
      frame False {
        n1857 = local read "stopT"() -> (w2803:bool)
        n1858 = case shown="True" w2803 {
          frame False {
          }
          frame True {
            n1859 = local write "stopT"(FALSE) -> ()
          }
        }
      }
      frame True {
        "stopT" <- TRUE
      }
    }
    n1860 = case shown="False" w1823 {
      frame False {
      }
      frame True {
      }
    }
    n1861 = case shown="True" w1813 {
      frame False {
        n1862 = property on="Password 2" class="Str"("Visible"=FALSE) -> ()  [unwired: 2 in, 2 out]
        n1863 = local write "Password 2"("" ("Password")) -> ()
      }
      frame True {
        n1864 = property on="Password 2" class="Str"("Visible"=TRUE) -> ()  [unwired: 2 in, 2 out]
        n1865 = Equal?(x="Password 2", y="HFRR1234") -> (x = y?=w1945:bool)
        n1866 = case shown="True" w1945 {
          tunnel: "Password 2" -> [w1948 _]
          frame False {
            n1867 = String Length(string=w1948) -> (length=w1949:i32)
            n1868 = Greater Than 0?(x=w1949) -> (x > 0?=w1947:bool)
            n1869 = case shown="False" w1947 {
              frame False {
                n1870 = property on="Password 2" class="Str"("Caption.Text"="Password (Advance Setting)") -> ()  [unwired: 2 in, 2 out]
              }
              frame True {
                n1871 = property on="Password 2" class="Str"("Caption.Text"="Incorrect Password!") -> ()  [unwired: 2 in, 2 out]
              }
            }
          }
          frame True {
            n1872 = local write "EDIT 2"(FALSE ("EDIT 2")) -> ()
            n1873 = local write "Password 2"("" ("Password")) -> ()
            n1874 = local write "Main Tab"(T2."Advance" ("Main Tab")) -> ()
            n1875 = local write "Main Dashboard Buttons"(T1."Advance" ("Main Dashboard Buttons")) -> ()
          }
        }
      }
    }
    n1876 = case shown="True" "Prog Uno" {
      frame False {
      }
      frame True {
        n1877 = stacked-sequence {
          frame #0 {
            n1878 = Delete(path (use dialog)=path "C:/LAB-IQ-NXT/UNOCOMPILE.bat" ("working directory")) -> ()  [unwired: 4 in, 3 out]
          }
          frame #1 {
            n1879 = local read "Com Port 1"() -> (w2410:refnum<visa-resource-name>)
            n1880 = Concatenate Strings("cmd.exe /c \"mode " ("command line"), w2410, ":1200,n,8,1\"\n" ("command line")) -> (w2415:string)
            n1881 = Concatenate Strings(w2415, "CD\\\nCD WinDucom\navrdude -C avrdude.conf -v -patmega328p -carduino -P" ("command line"), w2410, " -b115200 -D -Uflash:w:UNO_V20.hex:i\n" ("command line"), "\r") -> (w2417:string)
            "STR" <- w2417
            n1882 = call <vilib>:"Write Characters To File.vi"("append to file? (new file:F)"=FALSE, "character string"=w2417, "file path (dialog if empty)"=path "C:/LAB-IQ/UNOCOMPILE.bat" ("working directory")) -> ()  [unwired: 2 in, 1 out]
          }
          frame #2 {
            n1883 = disable-structure shown="Disabled" {
              frame Disabled {
                w2421 = "cmd.exe  /c \"C:\\LAB-IQ-NXT\\UNOCOMPILE.bat\"" ("string")
                n1884 = local write "Prog Uno"(FALSE ("run minimized? (F)")) -> ()
                n1885 = call <vilib>:"System Exec.vi"("expected output size  (4096)"=u32 65535, "run minimized? (F)"=FALSE, "wait until completion? (T)"=TRUE ("run minimized? (F)"), "working directory"=path "C:/LAB-IQ-NXT", "standard input"=w2421, "command line"=w2421) -> ("error out"=w2420:errorcluster, "standard output"=→"String 42":string)  [unwired: 2 in, 2 out]
                "error out 3" <- w2420
                n1886 = flat-sequence {
                  tunnel: w2420 -> [_]
                  frame #0 {
                  }
                }
              }
              frame Enabled {
              }
            }
          }
        }
      }
    }
    n1887 = case shown="\"ISO 12156\"" "TEST STANDARD" {
      tunnel: [2.0 ("Set Temp") 0.0 ("Set Temp") 2.0 ("Set Temp") 0.0 ("Set Temp")] -> w1814
      frame "ASTM D6079", Default {
        w2367 = 50.0 ("Hz")
        w2368 = 53.0 ("Set Rh")
        w2370 = 1.0 ("Set Strk")
        w2369 = 60.0 ("Set Temp")
        # "astm hide"
        n1888 = local write "NORMAL LOAD"(200.0 ("NORMAL LOAD")) -> ()
        n1889 = local write "Set Strk"(w2370) -> ()
        n1890 = local write "Set Hz"(w2367) -> ()
        n1891 = local write "Set Temp"(w2369) -> ()
        n1892 = local write "Set Rh"(w2368) -> ()
        n1893 = local write "test time"(75.0 ("test time")) -> ()
        n1894 = local write "Set Stroke:"(w2370) -> ()
        n1895 = local write "Set Humidity:"(w2368) -> ()
        n1896 = local write "Set Frequency:"(w2367) -> ()
        n1897 = local write "Set Temperature:"(w2369) -> ()
        "Test Standard" <- "ASTM D6079" ("Test Standard 2")
      }
      frame "ISO 12156" {
        n1898 = local write "Set Strk"(1.0 ("Set Strk")) -> ()
        n1899 = local write "NORMAL LOAD"(200.0 ("NORMAL LOAD")) -> ()
        n1900 = local write "Set Temp"(60.0 ("Set Temp")) -> ()
        n1901 = local write "test time"(75.0 ("test time")) -> ()
        n1902 = local write "Set Hz"(50.0 ("Hz")) -> ()
        n1903 = local write "Set Rh"(53.0 ("Set Rh")) -> ()
      }
      frame "CEC F-096-A-06" {
        n1904 = local write "Set Strk"(1.0 ("Set Strk")) -> ()
        n1905 = local write "NORMAL LOAD"(200.0 ("NORMAL LOAD")) -> ()
        n1906 = local write "Set Temp"(60.0 ("Set Temp")) -> ()
        n1907 = local write "test time"(75.0 ("test time")) -> ()
        n1908 = local write "Set Hz"(50.0 ("Hz")) -> ()
        n1909 = local write "Set Rh"(53.0 ("Set Rh")) -> ()
      }
      frame "Custom" {
      }
    }
    n1910 = case shown="True" "Prog Due" {
      frame False {
      }
      frame True {
        n1911 = stacked-sequence {
          frame #0 {
            n1912 = Delete(path (use dialog)=path "C:/LAB-IQ/DUECOMPILE.bat" ("working directory")) -> ()  [unwired: 4 in, 3 out]
          }
          frame #1 {
            n1913 = disable-structure shown="Disabled" {
              frame Disabled {
                n1914 = local read "visa due"() -> (w2392:string)
                n1915 = Concatenate Strings("cmd.exe /c \"mode " ("command line"), w2392, ":1200,n,8,1\"\n" ("command line")) -> (w2397:string)
                n1916 = Concatenate Strings(w2397, "CD\\\nCD WinDucom\nTIMEOUT 1\n bossac.exe -i -d --port=" ("command line"), w2392, " -U false -e -w -v -b DUE.bin -R\n" ("command line"), "\r") -> (w2399:string)
                "concatenated string 2" <- w2399
                n1917 = call <vilib>:"Write Characters To File.vi"("append to file? (new file:F)"=FALSE, "character string"=w2399, "file path (dialog if empty)"=path "C:/LAB-IQ-NXT/DUECOMPILE.bat" ("working directory")) -> ()  [unwired: 2 in, 1 out]
              }
              frame Enabled {
              }
            }
          }
          frame #2 {
            # "C:\\LAB-IQ-NXT\\DUECOMPILE.bat"
            n1918 = disable-structure shown="Disabled" {
              frame Disabled {
                w2404 = "cmd.exe  /c \"C:\\LAB-IQ-NXT\\DUECOMPILE.bat\"" ("string")
                n1919 = call <vilib>:"System Exec.vi"("expected output size  (4096)"=u32 65535, "run minimized? (F)"=FALSE, "wait until completion? (T)"=TRUE ("run minimized? (F)"), "working directory"=path "C:/LAB-IQ-NXT", "standard input"=w2404, "command line"=w2404) -> ("error out"=w2403:errorcluster, "standard output"=→"String 44":string)  [unwired: 2 in, 2 out]
                "error out 4" <- w2403
                n1920 = flat-sequence {
                  tunnel: w2403 -> [_]
                  frame #0 {
                  }
                }
              }
              frame Enabled {
              }
            }
            n1921 = local write "Prog Due"(FALSE ("Prog Due")) -> ()
          }
        }
      }
    }
    n1922 = Or(x=w1811, y=w1809) -> (x .or. y?=w1810:bool)
    n1923 = case shown="\"About\"" w1808 {
      tunnel: [T26."Acquire" ("Main Tab") T26."Compare Files" ("Main Tab") T26."About" ("Main Tab")] -> w1821
      frame "Acquire", Default {
      }
      frame "Compare Files" {
      }
      frame "About" {
      }
    }
    n1924 = Or(x=w1815, y="OPEN") -> (x .or. y?=w1816:bool)
    n1925 = case shown="True" w1816 {
      tunnel: w1815 -> [_ w1956]
      frame False {
      }
      frame True {
        n1926 = stacked-sequence {
          tunnel: w1956 -> [_ w2023 _ _]
          frame #0 {
            w1972 = "  " ("String 6")
            n1927 = local write "OPEN"(FALSE ("open")) -> ()
            n1928 = local read "string1 2"() -> (w1960:string)
            n1929 = local read "string1 3"() -> (w1959:string)
            n1930 = local read "string1 4"() -> (w1958:string)
            n1931 = property on="OPEN" class="Bool (strict)"("Visible"=FALSE) -> ()  [unwired: 2 in, 2 out]
            n1932 = local write "String 6"(w1972) -> ()
            n1933 = local write "String 7"(w1972) -> ()
            n1934 = local write "String 8"(w1972) -> ()
            n1935 = local write "String 12"(w1972) -> ()
            n1936 = local read "OK Button 16"() -> (w1957:bool)
            n1937 = String To Path(string=w1960) -> (path=w1968:path)
            n1938 = String To Path(string=w1959) -> (path=w1967:path)
            n1939 = String To Path(string=w1958) -> (path=w1966:path)
            n1940 = case shown="True" w1957 {
              tunnel: [w1973 w1974] -> w1961
              frame False {
                n1941 = local read "string1"() -> (w1973:string)
              }
              frame True {
                n1942 = local read "String Indicator 4"() -> (w1974:string)
              }
            }
            n1943 = Open/Create/Replace File "Open File"(file path (use dialog)=w1968) -> (refnum out=w1964:refnum<file>)  [unwired: 5 in, 2 out]
            n1944 = Open/Create/Replace File "Open File"(file path (use dialog)=w1967) -> (refnum out=w1963:refnum<file>)  [unwired: 5 in, 2 out]
            n1945 = Open/Create/Replace File "Open File"(file path (use dialog)=w1966) -> (refnum out=w1962:refnum<file>)  [unwired: 5 in, 2 out]
            n1946 = while {
              tunnel: w1964 -> [w1986]
              i -> [w1982]
              stop <- w1981 continue-if-true
              (unwired) TRUE ("line mode (F)")
              n1947 = Read from Text File "Read File"(file (use dialog)=w1986) -> (text=w1983:string)  [unwired: 3 in, 3 out]
              n1948 = local write "Numeric 11"(w1982) -> ()
              n1949 = String Length(string=w1983) -> (length=w1985:i32)
              n1950 = Greater?(x=w1985, y=1) -> (0:w1981:bool)
            }
            n1951 = while {
              tunnel: w1963 -> [w1992]
              i -> [w1988]
              stop <- w1987 continue-if-true
              (unwired) TRUE ("line mode (F)")
              n1952 = Read from Text File "Read File"(file (use dialog)=w1992) -> (text=w1989:string)  [unwired: 3 in, 3 out]
              n1953 = local write "Numeric 12"(w1988) -> ()
              n1954 = String Length(string=w1989) -> (length=w1991:i32)
              n1955 = Greater?(x=w1991, y=1) -> (0:w1987:bool)
            }
            n1956 = while {
              tunnel: w1962 -> [w1998]
              i -> [w1994]
              stop <- w1993 continue-if-true
              (unwired) TRUE ("line mode (F)")
              n1957 = Read from Text File "Read File"(file (use dialog)=w1998) -> (text=w1995:string)  [unwired: 3 in, 3 out]
              n1958 = local write "Numeric 13"(w1994) -> ()
              n1959 = String Length(string=w1995) -> (length=w1997:i32)
              n1960 = Greater?(x=w1997, y=1) -> (0:w1993:bool)
            }
            n1961 = String To Path(string=w1961) -> (path=w1969:path)
            n1962 = Open/Create/Replace File "Open File"(file path (use dialog)=w1969) -> (refnum out=w1965:refnum<file>)  [unwired: 5 in, 2 out]
            n1963 = while {
              tunnel: w1965 -> [w1980]
              i -> [w1976]
              stop <- w1975 continue-if-true
              (unwired) TRUE ("line mode (F)")
              n1964 = Read from Text File "Read File"(file (use dialog)=w1980) -> (text=w1977:string)  [unwired: 3 in, 3 out]
              n1965 = local write "Numeric 8"(w1976) -> ()
              n1966 = String Length(string=w1977) -> (length=w1979:i32)
              n1967 = Greater?(x=w1979, y=1) -> (0:w1975:bool)
            }
          }
          frame #1 {
            w2150 = FALSE ("ACTUAL   MERGE")
            # "Sample Temp"
            # "ECR"
            # "COF"
            # "Time\nCOF\nFF\nTemp"
            n1968 = case shown="True" w2023 {
              tunnel: [w2170 w2171] -> w2024
              frame False {
                n1969 = local read "string1"() -> (w2170:string)
              }
              frame True {
                n1970 = local read "String Indicator 4"() -> (w2171:string)
              }
            }
            n1971 = local read "string1 3"() -> (w2068:string)
            n1972 = String To Path(string=w2024) -> (path=w2155:path)
            n1973 = String To Path(string=w2068) -> (path=w2166:path)
            n1974 = local read "Numeric 12"() -> (w2152:i32)
            n1975 = local read "Numeric 8"() -> (w2154:i32)
            n1976 = local read "string1 2"() -> (w2069:string)
            n1977 = local read "string1 4"() -> (w2067:string)
            n1978 = Open/Create/Replace File "Open File"(file path (use dialog)=w2155) -> (refnum out=w2169:refnum<file>, error out=w2168:errorcluster)  [unwired: 5 in, 1 out]
            n1979 = Open/Create/Replace File "Open File"(file path (use dialog)=w2166) -> (refnum out=w2162:refnum<file>, error out=w2163:errorcluster)  [unwired: 5 in, 1 out]
            n1980 = for {
              N: w2154 -> [_]
              tunnel: w2169 -> [w2317]
              tunnel: w2168 -> [w2316]
              tunnel: [w2306] -> w2081 mode=indexing
              tunnel: [w2304] -> w2138 mode=indexing
              tunnel: [w2305] -> w2133 mode=indexing
              tunnel: w2150 -> [_]
              tunnel: [w2298] -> w2135 mode=indexing
              tunnel: [w2294] -> w2104 mode=indexing
              tunnel: [w2290] -> w2079 mode=indexing
              tunnel: [w2286] -> w2060 mode=indexing
              tunnel: [w2281] -> w2020 mode=indexing
              (unwired) TRUE ("line mode (F)")
              # "freq"
              # "Stroke"
              # "Time"
              # "CoF"
              # "Humidity"
              # "Temp"
              # "Air Temp"
              # "ECR"
              n1981 = Read from Text File "Read File"(file (use dialog)=w2317, error in=w2316) -> (text=w2282:string)  [unwired: 2 in, 3 out]
              n1982 = local write "String 6"(w2282) -> ()
              n1983 = String Subset(string=w2282, offset (0)=0, length (rest)=14 ("length (rest)")) -> (substring=w2310:string)
              n1984 = String Subset(string=w2282, offset (0)=35, length (rest)=9 ("length (rest)")) -> (substring=w2307:string)
              n1985 = String Subset(string=w2282, offset (0)=15, length (rest)=9 ("length (rest)")) -> (substring=w2313:string)
              n1986 = Fract/Exp String To Number(string=w2310) -> (number=w2306:dbl)  [unwired: 3 in, 1 out]
              n1987 = Fract/Exp String To Number(string=w2307) -> (number=w2305:dbl)  [unwired: 3 in, 1 out]
              n1988 = Fract/Exp String To Number(string=w2313) -> (number=w2304:dbl)  [unwired: 3 in, 1 out]
              n1989 = String Subset(string=w2282, offset (0)=85, length (rest)=9 ("length (rest)")) -> (substring=w2283:string)
              n1990 = String Subset(string=w2282, offset (0)=25, length (rest)=9 ("length (rest)")) -> (substring=w2289:string)
              n1991 = String Subset(string=w2282, offset (0)=55, length (rest)=9 ("length (rest)")) -> (substring=w2291:string)
              n1992 = String Subset(string=w2282, offset (0)=45, length (rest)=9 ("length (rest)")) -> (substring=w2297:string)
              n1993 = String Subset(string=w2282, offset (0)=65, length (rest)=9 ("length (rest)")) -> (substring=w2303:string)
              n1994 = Fract/Exp String To Number(string=w2289) -> (number=w2286:dbl)  [unwired: 3 in, 1 out]
              n1995 = Fract/Exp String To Number(string=w2283) -> (number=w2281:dbl)  [unwired: 3 in, 1 out]
              n1996 = Fract/Exp String To Number(string=w2291) -> (number=w2290:dbl)  [unwired: 3 in, 1 out]
              n1997 = Fract/Exp String To Number(string=w2297) -> (number=w2294:dbl)  [unwired: 3 in, 1 out]
              n1998 = Fract/Exp String To Number(string=w2303) -> (number=w2300:dbl)  [unwired: 3 in, 1 out]
              n1999 = Add(x=w2300, y=0.0) -> (x+y=w2298:dbl)
            }
            n2000 = for {
              N: w2152 -> [_]
              tunnel: w2163 -> [w2243]
              tunnel: w2162 -> [w2242]
              tunnel: [w2232] -> w2121 mode=indexing
              tunnel: [w2230] -> w2119 mode=indexing
              tunnel: [w2231] -> w2115 mode=indexing
              tunnel: w2150 -> [_]
              tunnel: [w2224] -> w2117 mode=indexing
              tunnel: [w2220] -> w2099 mode=indexing
              tunnel: [w2216] -> w2075 mode=indexing
              tunnel: [w2213] -> w2056 mode=indexing
              tunnel: [w2209] -> w2015 mode=indexing
              (unwired) 9 ("length (rest)")
              (unwired) 9 ("length (rest)")
              (unwired) TRUE ("line mode (F)")
              n2001 = Read from Text File "Read File"(file (use dialog)=w2242, error in=w2243) -> (text=w2210:string)  [unwired: 2 in, 3 out]
              n2002 = local write "String 8"(w2210) -> ()
              n2003 = String Subset(string=w2210, offset (0)=85) -> (substring=w2212:string)  [unwired: 1 in]
              n2004 = String Subset(string=w2210, offset (0)=35, length (rest)=9 ("length (rest)")) -> (substring=w2233:string)
              n2005 = String Subset(string=w2210, offset (0)=55, length (rest)=9 ("length (rest)")) -> (substring=w2218:string)
              n2006 = String Subset(string=w2210, offset (0)=25) -> (substring=w2214:string)  [unwired: 1 in]
              n2007 = String Subset(string=w2210, offset (0)=15, length (rest)=9 ("length (rest)")) -> (substring=w2239:string)
              n2008 = String Subset(string=w2210, offset (0)=0, length (rest)=14 ("length (rest)")) -> (substring=w2236:string)
              n2009 = String Subset(string=w2210, offset (0)=45, length (rest)=9 ("length (rest)")) -> (substring=w2223:string)
              n2010 = String Subset(string=w2210, offset (0)=65, length (rest)=9 ("length (rest)")) -> (substring=w2229:string)
              n2011 = Fract/Exp String To Number(string=w2212) -> (number=w2209:dbl)  [unwired: 3 in, 1 out]
              n2012 = Fract/Exp String To Number(string=w2233) -> (number=w2231:dbl)  [unwired: 3 in, 1 out]
              n2013 = Fract/Exp String To Number(string=w2218) -> (number=w2216:dbl)  [unwired: 3 in, 1 out]
              n2014 = Fract/Exp String To Number(string=w2214) -> (number=w2213:dbl)  [unwired: 3 in, 1 out]
              n2015 = Fract/Exp String To Number(string=w2239) -> (number=w2230:dbl)  [unwired: 3 in, 1 out]
              n2016 = Fract/Exp String To Number(string=w2236) -> (number=w2232:dbl)  [unwired: 3 in, 1 out]
              n2017 = Fract/Exp String To Number(string=w2223) -> (number=w2220:dbl)  [unwired: 3 in, 1 out]
              n2018 = Fract/Exp String To Number(string=w2229) -> (number=w2226:dbl)  [unwired: 3 in, 1 out]
              n2019 = Add(x=w2226, y=0.0) -> (x+y=w2224:dbl)
            }
            n2020 = String To Path(string=w2069) -> (path=w2167:path)
            n2021 = String To Path(string=w2067) -> (path=w2161:path)
            n2022 = local read "Numeric 11"() -> (w2151:i32)
            n2023 = local read "Numeric 13"() -> (w2153:i32)
            n2024 = Open/Create/Replace File "Open File"(file path (use dialog)=w2167) -> (refnum out=w2165:refnum<file>, error out=w2164:errorcluster)  [unwired: 5 in, 1 out]
            n2025 = Open/Create/Replace File "Open File"(file path (use dialog)=w2161) -> (refnum out=w2160:refnum<file>, error out=w2159:errorcluster)  [unwired: 5 in, 1 out]
            n2026 = for {
              N: w2151 -> [_]
              tunnel: w2165 -> [w2280]
              tunnel: w2164 -> [w2279]
              tunnel: [w2269] -> w2131 mode=indexing
              tunnel: [w2267] -> w2129 mode=indexing
              tunnel: [w2268] -> w2124 mode=indexing
              tunnel: w2150 -> [_]
              tunnel: [w2261] -> w2126 mode=indexing
              tunnel: [w2257] -> w2102 mode=indexing
              tunnel: [w2253] -> w2077 mode=indexing
              tunnel: [w2249] -> w2058 mode=indexing
              tunnel: [w2244] -> w2016 mode=indexing
              (unwired) TRUE ("line mode (F)")
              n2027 = Read from Text File "Read File"(file (use dialog)=w2280, error in=w2279) -> (text=w2245:string)  [unwired: 2 in, 3 out]
              n2028 = local write "String 7"(w2245) -> ()
              n2029 = String Subset(string=w2245, offset (0)=85, length (rest)=9 ("length (rest)")) -> (substring=w2248:string)
              n2030 = String Subset(string=w2245, offset (0)=35, length (rest)=9 ("length (rest)")) -> (substring=w2270:string)
              n2031 = String Subset(string=w2245, offset (0)=55, length (rest)=9 ("length (rest)")) -> (substring=w2256:string)
              n2032 = String Subset(string=w2245, offset (0)=25, length (rest)=9 ("length (rest)")) -> (substring=w2250:string)
              n2033 = String Subset(string=w2245, offset (0)=45, length (rest)=9 ("length (rest)")) -> (substring=w2258:string)
              n2034 = String Subset(string=w2245, offset (0)=0, length (rest)=14 ("length (rest)")) -> (substring=w2273:string)
              n2035 = String Subset(string=w2245, offset (0)=15, length (rest)=9 ("length (rest)")) -> (substring=w2276:string)
              n2036 = String Subset(string=w2245, offset (0)=65, length (rest)=9 ("length (rest)")) -> (substring=w2262:string)
              n2037 = Fract/Exp String To Number(string=w2248) -> (number=w2244:dbl)  [unwired: 3 in, 1 out]
              n2038 = Fract/Exp String To Number(string=w2270) -> (number=w2268:dbl)  [unwired: 3 in, 1 out]
              n2039 = Fract/Exp String To Number(string=w2256) -> (number=w2253:dbl)  [unwired: 3 in, 1 out]
              n2040 = Fract/Exp String To Number(string=w2250) -> (number=w2249:dbl)  [unwired: 3 in, 1 out]
              n2041 = Fract/Exp String To Number(string=w2258) -> (number=w2257:dbl)  [unwired: 3 in, 1 out]
              n2042 = Fract/Exp String To Number(string=w2273) -> (number=w2269:dbl)  [unwired: 3 in, 1 out]
              n2043 = Fract/Exp String To Number(string=w2276) -> (number=w2267:dbl)  [unwired: 3 in, 1 out]
              n2044 = Fract/Exp String To Number(string=w2262) -> (number=w2265:dbl)  [unwired: 3 in, 1 out]
              n2045 = Add(x=w2265, y=0.0) -> (x+y=w2261:dbl)
            }
            n2046 = for {
              N: w2153 -> [_]
              tunnel: w2160 -> [w2208]
              tunnel: w2159 -> [w2207]
